vi "XML to TOC.vi"(7 "XML File Path":path=path "C:/Users/JMS/Documents/PDF Report/Essais pdf/outline_actions6.xml", 11 "error in (no error)":errorcluster) -> (4 "Type":T1=enum."ASCII", 8 "TOC [ ]":T2[](array[typedef])=[{"Title"="1. Introduction", "Level"=1, "GoTo Page"=2, "GoTo Position"=720, "Destination"="", "Type & run direction"=enum."Select"}, {"Title"="2. Installation", "Level"=1, "GoTo Page"=2, "GoTo Position"=480, "Destination"="", "Type & run direction"=enum."Select"}, {"Title"="3. PDF Report (simplified)", "Level"=1, "GoTo Page"=5, "GoTo Position"=720, "Destination"="", "Type & run direction"=enum."Select"}, {"Title"="4. General", "Level"=1, "GoTo Page"=6, "GoTo Position"=720, "Destination"="", "Type & run direction"=enum."Select"}, {"Title"="5. The different palettes", "Level"=1, "GoTo Page"=7, "GoTo Position"=720, "Destination"="", "Type & run direction"=enum."Select"}, {"Title"="5.1. The &quot;Text&quot; palette ", "Level"=2, "GoTo Page"=7, "GoTo Position"=702, "Destination"="", "Type & run direction"=enum."Select"}, {"Title"="5.2. The &quot;Image&quot; palette", "Level"=2, "GoTo Page"=11, "GoTo Position"=720, "Destination"="", "Type & run direction"=enum."Select"}, {"Title"="5.3. The &quot;Table&quot; palette", "Level"=2, "GoTo Page"=14, "GoTo Position"=720, "Destination"="", "Type & run direction"=enum."Select"}, {"Title"="5.4. The &quot;Document&quot; palette", "Level"=2, "GoTo Page"=23, "GoTo Position"=720, "Destination"="", "Type & run direction"=enum."Select"}, {"Title"="5.5. Header, Footer and Watermark palette", "Level"=2, "GoTo Page"=27, "GoTo Position"=660, "Destination"="", "Type & run direction"=enum."Select"}, {"Title"="5.6. The &quot;Concatenate&quot; palette", "Level"=2, "GoTo Page"=33, "GoTo Position"=720, "Destination"="", "Type & run direction"=enum."Select"}, {"Title"="6. Unicode (UTF-16) with PDF Report", "Level"=1, "GoTo Page"=34, "GoTo Position"=720, "Destination"="", "Type & run direction"=enum."Select"}, {"Title"="7. Build application with error 1172", "Level"=1, "GoTo Page"=36, "GoTo Position"=720, "Destination"="", "Type & run direction"=enum."Select"}], 15 "error out":errorcluster)   [LabVIEW 2019]
doc: "Version 1.1\nDeveloped by Jean-Marc Simard\nCopyright © 2012, Exaprom Inc.\nAll rights reserved.\nLicense: BSD\n\nWith iTextSharp 4.1.6 (http://itextsharp.sourceforge.net)\nunder Mozilla Public License Version 1.1\n(http://www.mozilla.org/MPL/MPL-1.1.html)"
uses:
  <userlib>/Exaprom PDF/Controls/Text Controls/Unicode/Character type with Select.ctl
  <userlib>/Exaprom PDF/Controls/Chapter Controls/TOC Line.ctl
  <userlib>/Exaprom PDF/Controls/Text Controls/Unicode/Type and run direction.ctl
panel:
  out "text":string
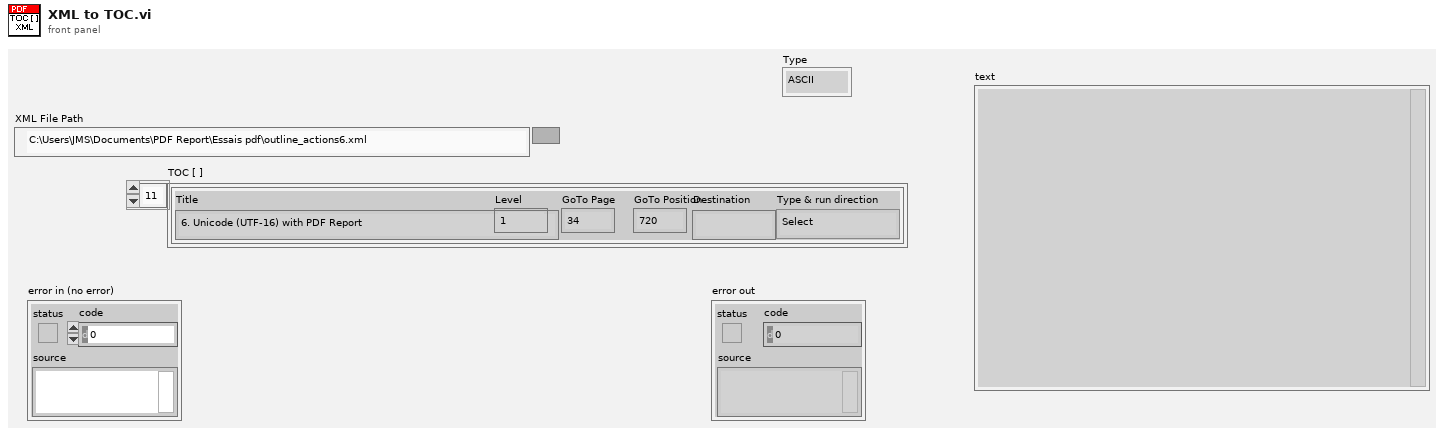
[diagram p1: front panel]
types:
  T1 = typedef "Character type with Select.ctl" = enum16{"Select", "ASCII", "Unicode"}
  T2 = typedef "TOC Line.ctl" = cluster{"Title":string, "Level":u16, "GoTo Page":u16, "GoTo Position":u16, "Destination":string, "Type & run direction":T3}
  T3 = typedef "Type and run direction.ctl" = enum16{"Select", "ASCII", "UTF-16", "UTF-16 (default)", "UTF-16 (LTR)", "UTF-16 (RTL)"}
  T4 = cluster{string, "number of replacements":i32, i32, i32, string, "Type":T1}
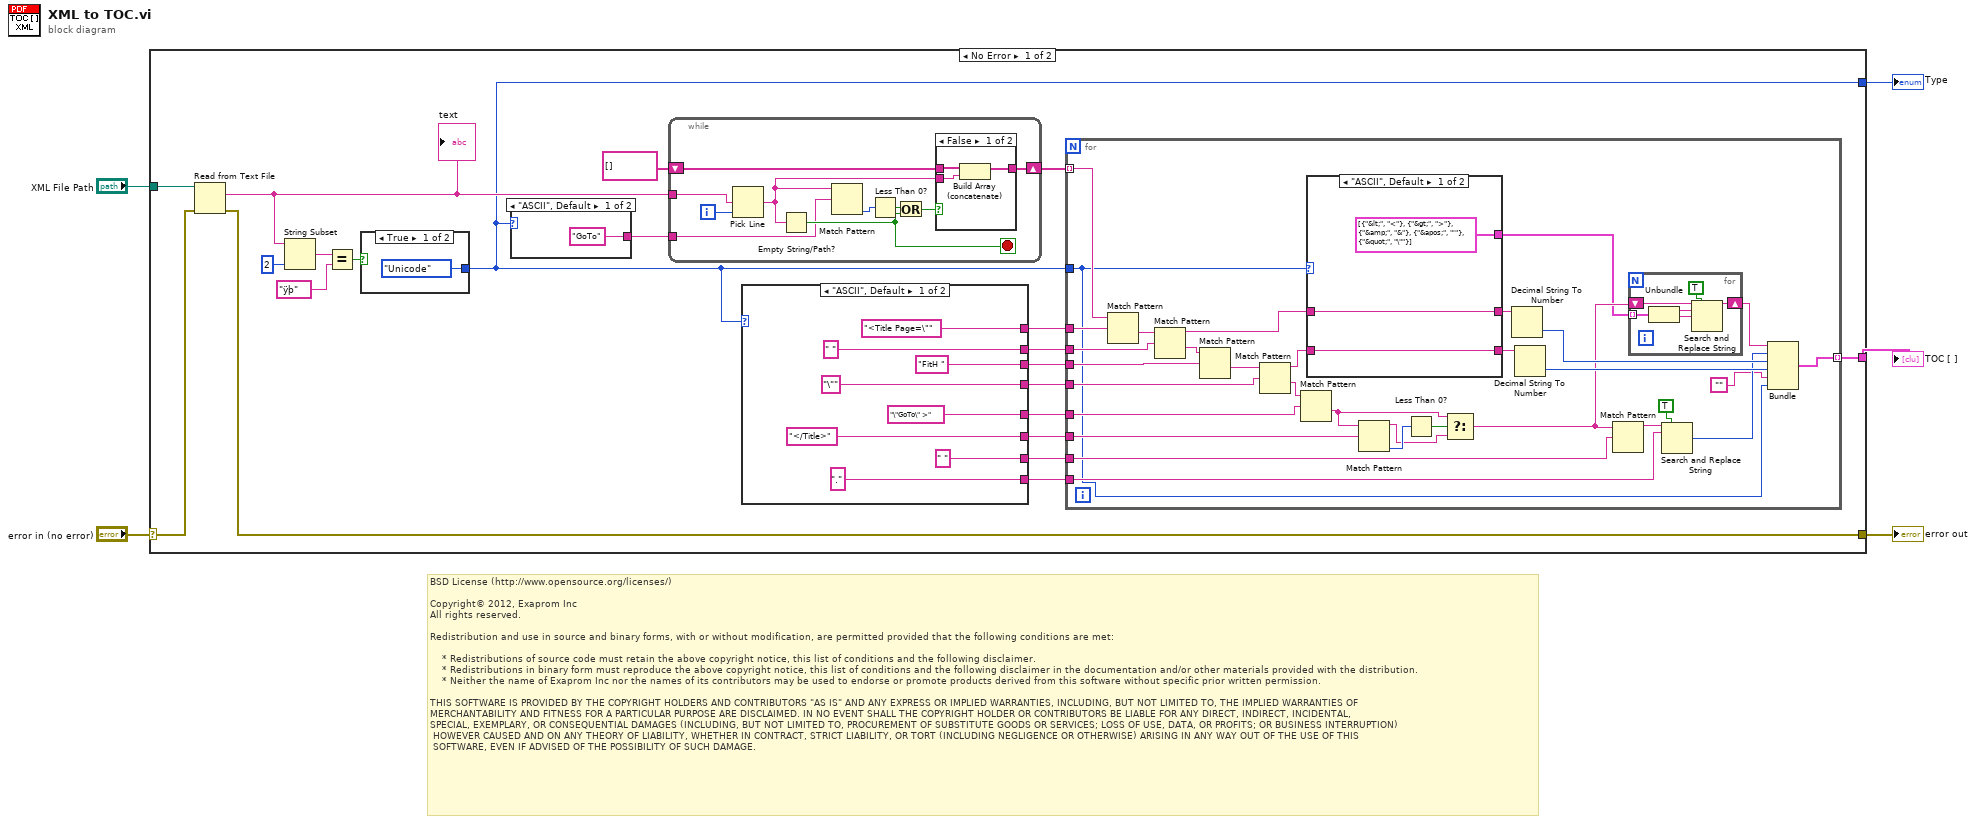
[diagram p0: block diagram]
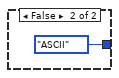
[diagram p2: hidden frame]
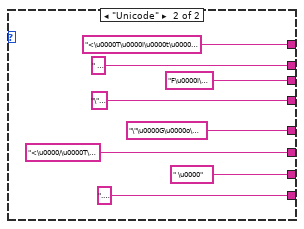
[diagram p3: hidden frame]
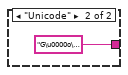
[diagram p4: hidden frame]
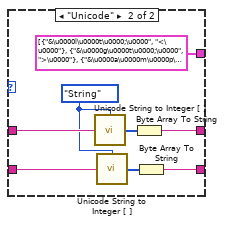
[diagram p5: hidden frame]
diagram:
  # "BSD License (http://www.opensource.org/licenses/)\n\nCopyright© 2012, Exaprom Inc\nAll rights reserved.\n\nRedistribution and use in source and binary forms, with or without modification, are permitted provided that the following conditions are met:\n\n    * Redistributions of source code must retain the above copyright notice, this list of conditions and the following disclaimer.\n    * Redistributions in binary form must reproduce the above copyright notice, this list of conditions and the following disclaimer in the documentation and/or other materials provided with the distribution.\n    * Neither the name of Exaprom Inc nor the names of its contributors may be used to endorse or promote products derived from this software without specific prior written permission.\n\nTHIS SOFTWARE IS PROVIDED BY THE COPYRIGHT HOLDERS AND CONTRIBUTORS \"AS IS\" AND ANY EXPRESS OR IMPLIED WARRANTIES, INCLUDING, BUT NOT LIMITED TO, THE IMPLIED WARRANTIES OF \nMERCHANTABILITY AND FITNESS FOR A PARTICULAR PURPOSE ARE DISCLAIMED. IN NO EVENT SHALL THE COPYRIGHT HOLDER OR CONTRIBUTORS BE LIABLE FOR ANY DIRECT, INDIRECT, INCIDENTAL,\nSPECIAL, EXEMPLARY, OR CONSEQUENTIAL DAMAGES (INCLUDING, BUT NOT LIMITED TO, PROCUREMENT OF SUBSTITUTE GOODS OR SERVICES; LOSS OF USE, DATA, OR PROFITS; OR BUSINESS INTERRUPTION)\n HOWEVER CAUSED AND ON ANY THEORY OF LIABILITY, WHETHER IN CONTRACT, STRICT LIABILITY, OR TORT (INCLUDING NEGLIGENCE OR OTHERWISE) ARISING IN ANY WAY OUT OF THE USE OF THIS\n SOFTWARE, EVEN IF ADVISED OF THE POSSIBILITY OF SUCH DAMAGE."
  n1 = case shown="No Error" "error in (no error)" {
    selector: "error in (no error)" -> [w10 w110]
    tunnel: [w9 w110] -> w5
    tunnel: "XML File Path" -> [w8 _]
    tunnel: [w7 _] -> w2
    tunnel: [w6 _] -> w1
    frame No Error {
      n2 = Read from Text File(file (use dialog)=w8, error in=w10) -> (text=w23:string, error out=w9:errorcluster)  [unwired: 2 in, 2 out]
      "text" <- w23
      n3 = String Subset(string=w23, length (rest)=2 ("offset (0)")) -> (substring=w24:string)  [unwired: 1 in]
      n4 = Equal?(x=w24, y="ÿþ") -> (x = y?=w26:bool)
      n5 = case shown="True" w26 {
        tunnel: [Character_type_with_Select."Unicode" ("Type") Character_type_with_Select."ASCII" ("Type")] -> w7
        frame True {
        }
        frame False {
        }
      }
      n6 = case shown="\"ASCII\", Default" w7 {
        tunnel: ["GoTo" ("regular expression") "G\u0000o\u0000T\u0000o\u0000"] -> w13
        frame "ASCII", Default {
        }
        frame "Unicode" {
        }
      }
      n7 = while {
        tunnel: w23 -> [w105]
        shift-right: [w102] -> w12
        shift-left: string[] [] -> [w103]
        tunnel: w13 -> [w96]
        i -> [w104]
        stop <- w98 stop-if-true
        n8 = Pick Line(multi-line string=w105, line index=w104) -> (output string=w101:string)  [unwired: 1 in]
        n9 = Empty String/Path?(string/path=w101) -> (empty?=w98:bool)
        n10 = Match Pattern(string=w101, regular expression=w96) -> (offset past match=w100:i32)  [unwired: 1 in, 3 out]
        n11 = Less Than 0?(x=w100) -> (x < 0?=w99:bool)
        n12 = Or(x=w99, y=w98) -> (x .or. y?=w97:bool)
        n13 = case shown="False" w97 {
          tunnel: w103 -> [w108 w109]
          tunnel: [w106 w109] -> w102
          tunnel: w101 -> [w107 _]
          frame False {
            n14 = Build Array (concatenate)(w108, w107) -> (w106:string[])
          }
          frame True {
          }
        }
      }
      n15 = case shown="\"ASCII\", Default" w7 {
        tunnel: ["<Title Page=\"" ("regular expression") "<\u0000T\u0000i\u0000t\u0000l\u0000e\u0000 \u0000P\u0000a\u0000g\u0000e\u0000=\u0000\"\u0000" ("regular expression")] -> w14
        tunnel: [" " ("regular expression") " \u0000" ("regular expression")] -> w15
        tunnel: ["FitH " ("regular expression") "F\u0000i\u0000t\u0000H\u0000 \u0000" ("regular expression")] -> w16
        tunnel: ["\"" ("regular expression") "\"\u0000" ("regular expression")] -> w17
        tunnel: ["\"GoTo\" >" ("regular expression") "\"\u0000G\u0000o\u0000T\u0000o\u0000\"\u0000 \u0000>\u0000" ("regular expression")] -> w18
        tunnel: ["</Title>" ("regular expression") "<\u0000/\u0000T\u0000i\u0000t\u0000l\u0000e\u0000>\u0000" ("regular expression")] -> w19
        tunnel: [" " ("regular expression") " \u0000" ("regular expression")] -> w20
        tunnel: ["." ("search string") ".\u0000" ("search string")] -> w21
        frame "ASCII", Default {
        }
        frame "Unicode" {
        }
      }
      n16 = for {
        tunnel: w12 -> [w78] mode=indexing
        tunnel: [w71] -> w6 mode=indexing
        tunnel: w14 -> [w61]
        tunnel: w15 -> [w60]
        tunnel: w16 -> [w59]
        tunnel: w17 -> [w58]
        tunnel: w18 -> [w57]
        tunnel: w19 -> [w56]
        tunnel: w20 -> [w55]
        tunnel: w21 -> [w54]
        tunnel: w7 -> [w47]
        n17 = Match Pattern(string=w78, regular expression=w61) -> (after substring=w70:string)  [unwired: 1 in, 3 out]
        n18 = Match Pattern(string=w70, regular expression=w60) -> (before substring=w53:string, after substring=w77:string)  [unwired: 1 in, 2 out]
        n19 = Match Pattern(string=w77, regular expression=w59) -> (after substring=w76:string)  [unwired: 1 in, 3 out]
        n20 = Match Pattern(string=w76, regular expression=w58) -> (before substring=w49:string, after substring=w75:string)  [unwired: 1 in, 2 out]
        n21 = Match Pattern(string=w75, regular expression=w57) -> (after substring=w65:string)  [unwired: 1 in, 3 out]
        n22 = case shown="\"ASCII\", Default" w47 {
          tunnel: w53 -> [w80 w88]
          tunnel: [w80 w87] -> w52
          tunnel: [w79 w85] -> w51
          tunnel: w49 -> [w79 w84]
          tunnel: [cluster{string, string}[] [{"&lt;", "<"}, {"&gt;", ">"}, {"&amp;", "&"}, {"&apos;", "'"}, {"&quot;", "\""}] cluster{string, string}[] [{"&\u0000l\u0000t\u0000;\u0000", "<\u0000"}, {"&\u0000g\u0000t\u0000;\u0000", ">\u0000"}, {"&\u0000a\u0000m\u0000p\u0000;\u0000", "&\u0000"}, {"&\u0000a\u0000p\u0000o\u0000s\u0000;\u0000", "'\u0000"}, {"&\u0000q\u0000u\u0000o\u0000t\u0000;\u0000", "\"\u0000"}]] -> w50
          frame "ASCII", Default {
          }
          frame "Unicode" {
            w83 = enum16{"String", "U16 [ ]"}."String" ("From")
            n23 = call <userlib>:"Unicode String to Integer [ ].vi"("From"=w83, "Unicode String"=w88) -> ("Char U16 [ ]"=w89:u16[])  [unwired: 11 in, 2 out]
            n24 = call <userlib>:"Unicode String to Integer [ ].vi"("From"=w83, "Unicode String"=w84) -> ("Char U16 [ ]"=w86:u16[])  [unwired: 11 in, 2 out]
            n25 = Byte Array To String(unsigned byte array=w89) -> (string=w87:string)
            n26 = Byte Array To String(unsigned byte array=w86) -> (string=w85:string)
          }
        }
        n27 = Match Pattern(string=w65, regular expression=w56) -> (before substring=w64:string, offset past match=w74:i32)  [unwired: 1 in, 2 out]
        n28 = Less Than 0?(x=w74) -> (x < 0?=w73:bool)
        n29 = Select(t=w65, s=w73, f=w64) -> (s? t:f=w63:string)
        n30 = Decimal String To Number(string=w52) -> (number=w69:i32)  [unwired: 2 in, 1 out]
        n31 = Decimal String To Number(string=w51) -> (number=w72:i32)  [unwired: 2 in, 1 out]
        n32 = Match Pattern(string=w63, regular expression=w55) -> (before substring=w68:string)  [unwired: 1 in, 3 out]
        n33 = for {
          shift-right: [w95] -> w62
          shift-left: w63 -> [w94]
          tunnel: w50 -> [w92] mode=indexing
          n34 = Unbundle(w92) -> (w93:string, w91:string)
          n35 = Search and Replace String(replace all?=TRUE ("replace all? (F)"), input string=w94, search string=w93, replace string=w91) -> (result string=w95:string)  [unwired: 4 in, 3 out]
        }
        n36 = Search and Replace String(replace all?=TRUE ("replace all? (F)"), input string=w68, search string=w54) -> (number of replacements=w67:i32)  [unwired: 5 in, 3 out]
        n37 = Bundle(w62, "number of replacements"=w67, w69, w72, "", "Type"=w47) -> (w71:T4)  [unwired: 1 in]
      }
    }
    frame Error {
    }
  }
  "error out" <- w5
  "Type" <- w2
  "TOC [ ]" <- w1
